vi "Test Hardware Manager.vi"() -> ()   [LabVIEW 2020]
uses:
  Classes/Communications/Server/Base Server/Server.lvclass
  HardwareManager/HardwareManager.lvclass
  C:/TestSystemServices/Total Fire Systems/Main/Tree/Classes/Service/Service.lvclass
  Hardware Components/Instrument/Instrument.lvclass
  User Interfaces/QControls/HardwareManagerUI/HardwareManagerUI.lvclass
  Classes/Service/Service.lvclass
panel:
  in  "UI":cluster{"ComboBox":string}
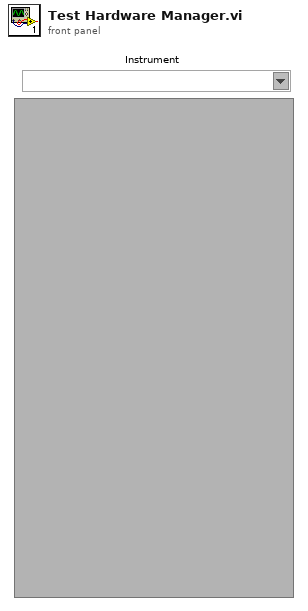
[diagram p1: front panel]
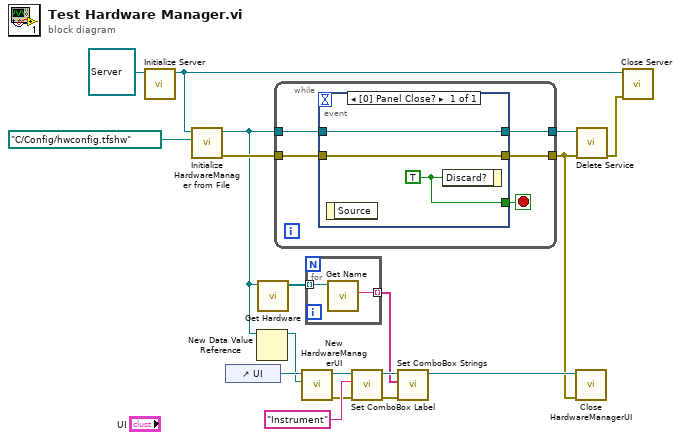
[diagram p0: block diagram]
diagram:
  n1 = call-dynamic "Initialize Server.vi"("Base Server in"=refnum<class "Server.lvclass"> refnum ("Server.lvclass")) -> ("Base Server out"=w5:refnum<class "Server.lvclass">)  [unwired: 9 in, 1 out]
  n2 = call "Initialize HardwareManager from File.vi"("Hardware Config Filepath"=path "C:/Config/hwconfig.tfshw", "Server in"=w5) -> ("error out"=w4:errorcluster, "HardwareManager out"=w2:refnum<class "HardwareManager.lvclass">)  [unwired: 8 in]
  n3 = control-ref of="UI"() -> (w17:refnum<vi>)
  n4 = New Data Value Reference(data value=w2) -> (data value reference=w16:refnum<data-value>)  [unwired: 1 in, 1 out]
  n5 = call "Get Hardware.vi"("Template Service in"=w2) -> ("Instruments"=w3:refnum<class "Instrument.lvclass">[])  [unwired: 9 in, 1 out]
  n6 = while {
    tunnel: w4 -> [w23]
    tunnel: [w21] -> w7
    tunnel: [w20] -> w9
    tunnel: w2 -> [w19]
    stop <- w22 stop-if-true
    n7 = event shown="[0] Panel Close?" {
      selector: _ -> [_]
      dyn-events: _ -> [_]
      timeout: _ -> [_]
      tunnel: w23 -> [w25]
      tunnel: [w26] -> w22
      tunnel: [w25] -> w21
      tunnel: [w24] -> w20
      tunnel: w19 -> [w24]
      event Panel Close? {
        w26 = TRUE ("Discard?")
        n8 = event-data() -> ()  [unwired: 1 in, 1 out]
        n9 = event-data("Discard?"=w26) -> ()  [unwired: 1 in, 1 out]
      }
    }
  }
  n10 = call "New HardwareManagerUI.vi"("HW Manager Ref"=w16, "Reference"=w17) -> ("error out"=w11:errorcluster, "HardwareManagerUI out"=w15:refnum<class "HardwareManagerUI.lvclass">)  [unwired: 8 in]
  n11 = for {
    tunnel: w3 -> [w28] mode=indexing
    tunnel: [w27] -> w1 mode=indexing
    n12 = call "Get Name.vi"("Service in"=w28) -> ("Name"=w27:string)  [unwired: 8 in, 2 out]
  }
  n13 = call "Set ComboBox Label.vi"("error in (no error)"=w11, "Label"="Instrument", "HardwareManagerUI in"=w15) -> ("error out"=w12:errorcluster, "HardwareManagerUI out"=w13:refnum<class "HardwareManagerUI.lvclass">)  [unwired: 7 in]
  n14 = call "Set ComboBox Strings.vi"("error in (no error)"=w12, "Names"=w1, "HardwareManagerUI in"=w13) -> ("HardwareManagerUI out"=w10:refnum<class "HardwareManagerUI.lvclass">)  [unwired: 7 in, 1 out]
  n15 = call "Close HardwareManagerUI.vi"("error in (no error)"=w7, "HardwareManagerUI in"=w10) -> ()  [unwired: 9 in, 1 out]
  n16 = call "Delete Service.vi"("error in (no error)"=w7, "Service in"=w9) -> ("error out"=w8:errorcluster)  [unwired: 9 in]
  n17 = call-dynamic "Close Server.vi"("error in (no error)"=w8, "Base Server in"=w5) -> ()  [unwired: 8 in, 2 out]
